vi "Create DFS Maze.vi"(10 "Height":i32, 11 "Width":i32) -> (3 "Maze":refnum<class "Maze.lvclass">)   [LabVIEW 2020, in "Maze.lvlib" / "MazeGen.lvclass"]
uses:
  MazeGen.lvclass
  Maze/Maze.lvclass
  Adjacency.ctl
  Position.ctl
  Maze.lvlib
panel:
  out "Preview":T1[][](array[typedef])
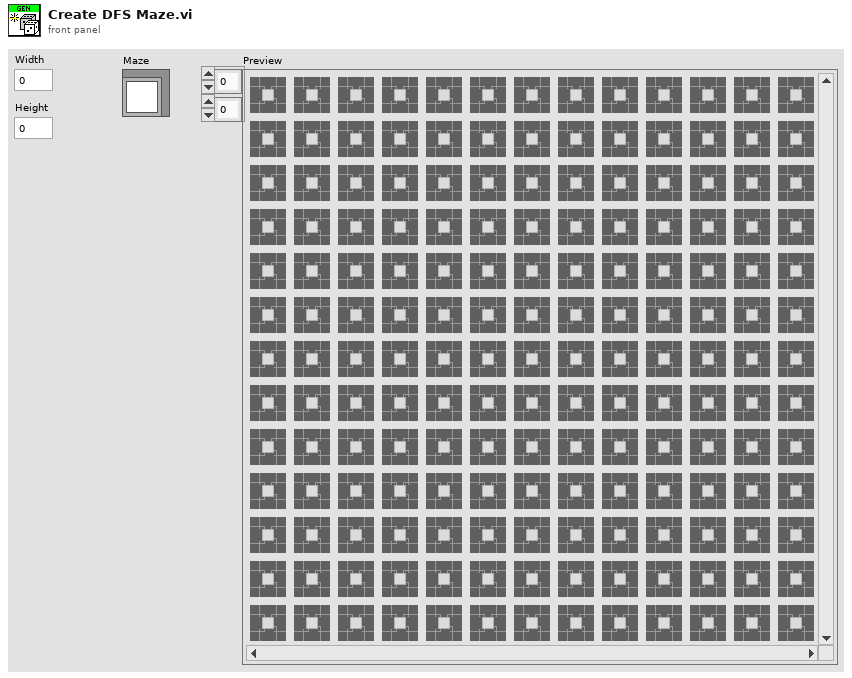
[diagram p1: front panel]
types:
  T1 = typedef "Maze.lvlib/Adjacency.ctl" = cluster{"E":bool, "N":bool, "W":bool, "S":bool, "Goal":bool, "Start":bool}
  T2 = typedef "Maze.lvlib/Position.ctl" = cluster{"S":i32, "E":i32}
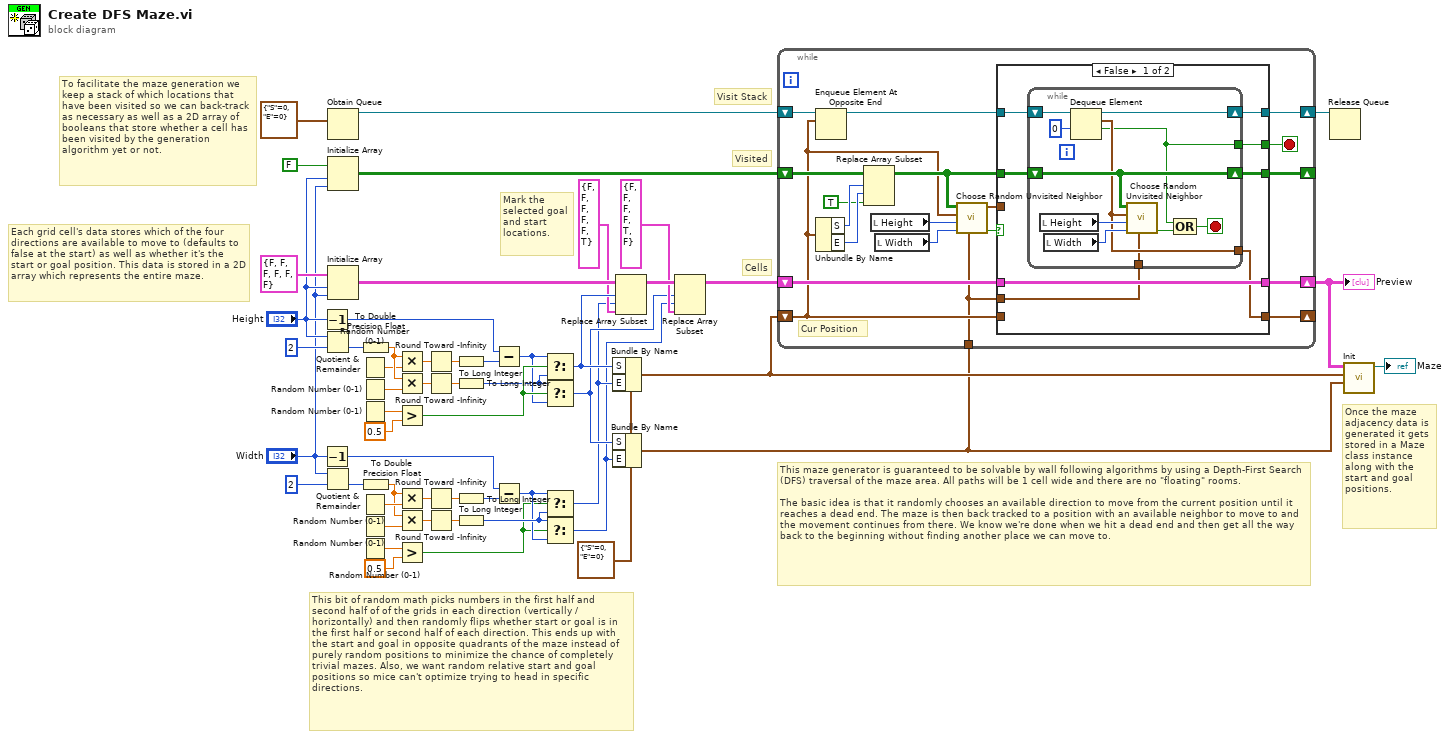
[diagram p0: block diagram]
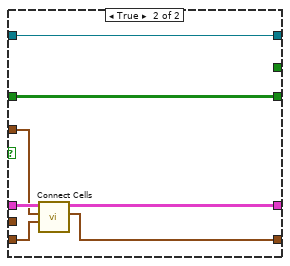
[diagram p2: hidden frame]
diagram:
  w26 = T2 {"S"=0, "E"=0} ("Position")
  # "Once the maze adjacency data is generated it gets stored in a Maze class instance along with the start and goal positions."
  # "Mark the selected goal and start locations."
  # "To facilitate the maze generation we keep a stack of which locations that have been visited so we can back-track as necessary as well as a 2D array of booleans that store whether a cell has been visited by the generation algorithm yet or not."
  # "Each grid cell's data stores which of the four directions are available to move to (defaults to false at the start) as well as whether it's the start or goal position. This data is stored in a 2D array which represents the entire maze."
  # "This maze generator is guaranteed to be solvable by wall following algorithms by using a Depth-First Search (DFS) traversal of the maze area. All paths will be 1 cell wide and there are no \"floating\" rooms.\n\nThe basic idea is that it randomly chooses an available direction to move from the current position until it reaches a dead end. The maze is then back tracked to a position with an available neighbor to move to and the movement continues from there. We know we're done when we hit a dead end and then get all the way back to the beginning without finding another place we can move to."
  # "This bit of random math picks numbers in the first half and second half of of the grids in each direction (vertically / horizontally) and then randomly flips whether start or goal is in the first half or second half of each direction. This ends up with the start and goal in opposite quadrants of the maze instead of purely random positions to minimize the chance of completely trivial mazes. Also, we want random relative start and goal positions so mice can't optimize trying to head in specific directions."
  # "Visit Stack"
  # "Visited"
  # "Cells"
  n1 = Decrement(x="Height") -> (x-1=w34:i32)
  n2 = Decrement(x="Width") -> (x-1=w44:i32)
  n3 = Quotient & Remainder(x="Height", y=2) -> (floor(x/y)=w29:i32)  [unwired: 1 out]
  n4 = Quotient & Remainder(x="Width", y=2) -> (floor(x/y)=w52:i32)  [unwired: 1 out]
  n5 = Obtain Queue(element data type=T2 {"S"=0, "E"=0} ("Position")) -> (queue out=w16:refnum<queue>)  [unwired: 4 in, 2 out]
  n6 = Initialize Array(FALSE, "Height", "Width") -> (w15:bool[][])
  n7 = Initialize Array(T1 {"E"=FALSE, "N"=FALSE, "W"=FALSE, "S"=FALSE, "Goal"=FALSE, "Start"=FALSE} ("Adjacency"), "Height", "Width") -> (w10:T1[][])
  n8 = Random Number (0-1)() -> (number: 0 to 1=w30:dbl)
  n9 = Random Number (0-1)() -> (number: 0 to 1=w31:dbl)
  n10 = Random Number (0-1)() -> (number: 0 to 1=w35:dbl)
  n11 = Random Number (0-1)() -> (number: 0 to 1=w51:dbl)
  n12 = Random Number (0-1)() -> (number: 0 to 1=w50:dbl)
  n13 = Random Number (0-1)() -> (number: 0 to 1=w43:dbl)
  n14 = To Double Precision Float(number=w29) -> (double precision float=w32:dbl)
  n15 = To Double Precision Float(number=w52) -> (double precision float=w49:dbl)
  n16 = Multiply(x=w32, y=w30) -> (x*y=w22:dbl)
  n17 = Multiply(x=w32, y=w31) -> (x*y=w21:dbl)
  n18 = Greater?(x=w35, y=0.5) -> (0:w38:bool)
  n19 = Multiply(x=w49, y=w51) -> (x*y=w24:dbl)
  n20 = Multiply(x=w49, y=w50) -> (x*y=w46:dbl)
  n21 = Greater?(x=w43, y=0.5) -> (0:w39:bool)
  n22 = Round Toward -Infinity(1:w22) -> (0:w19:dbl)
  n23 = Round Toward -Infinity(1:w21) -> (0:w20:dbl)
  n24 = Round Toward -Infinity(1:w24) -> (0:w23:dbl)
  n25 = Round Toward -Infinity(1:w46) -> (0:w25:dbl)
  n26 = To Long Integer(number=w19) -> (32bit integer=w33:i32)
  n27 = To Long Integer(number=w20) -> (32bit integer=w36:i32)
  n28 = To Long Integer(number=w23) -> (32bit integer=w45:i32)
  n29 = To Long Integer(number=w25) -> (32bit integer=w41:i32)
  n30 = Subtract(x=w34, y=w33) -> (x-y=w37:i32)
  n31 = Subtract(x=w44, y=w45) -> (x-y=w40:i32)
  n32 = Select(t=w37, s=w38, f=w36) -> (s? t:f=w9:i32)
  n33 = Select(t=w36, s=w38, f=w37) -> (s? t:f=w5:i32)
  n34 = Select(t=w40, s=w39, f=w41) -> (s? t:f=w4:i32)
  n35 = Select(t=w41, s=w39, f=w40) -> (s? t:f=w2:i32)
  n36 = Bundle By Name(cluster=w26, "S"=w9, "E"=w4) -> (w12:T2)
  n37 = Bundle By Name(cluster=w26, "S"=w5, "E"=w2) -> (w1:T2)
  n38 = Replace Array Subset(array=w10, new element=T1 {"E"=FALSE, "N"=FALSE, "W"=FALSE, "S"=FALSE, "Goal"=FALSE, "Start"=TRUE} ("new element/subarray"), index (row)=w9, index (col)=w4) -> (w7:T1[][])
  n39 = Replace Array Subset(array=w7, new element=T1 {"E"=FALSE, "N"=FALSE, "W"=FALSE, "S"=FALSE, "Goal"=TRUE, "Start"=FALSE} ("new element/subarray"), index (row)=w5, index (col)=w2) -> (w3:T1[][])
  n40 = while {
    shift-right: [w61] -> _
    shift-left: w12 -> [w57]
    shift-right: [w58] -> w14
    shift-left: w16 -> [w69]
    shift-right: [w59] -> _
    shift-left: w15 -> [w73]
    shift-right: [w60] -> w13
    shift-left: w3 -> [w62]
    tunnel: w1 -> [w55]
    stop <- w56 stop-if-true
    # "Cur Position"
    n41 = Enqueue Element At Opposite End(queue=w69, element=w57) -> (queue out=w64:refnum<queue>)  [unwired: 2 in, 2 out]
    n42 = Unbundle By Name(w57) -> ("S"=w72:i32, "E"=w71:i32)
    n43 = Replace Array Subset(array=w73, new element=TRUE ("new element/subarray"), index (row)=w72, index (col)=w71) -> (w63:bool[][])
    n44 = local read "Height"() -> (w68:i32)
    n45 = local read "Width"() -> (w67:i32)
    n46 = call "Choose Random Unvisited Neighbor.vi"("Goal"=w55, "Width"=w67, "Height"=w68, "Position"=w57, "Visited"=w63) -> ("Valid?"=w66:bool, "Random Unvisited Neighbor"=w65:T2)  [unwired: 5 in]
    n47 = case shown="False" w66 {
      tunnel: w65 -> [_ w96]
      tunnel: w64 -> [w81 w93]
      tunnel: w63 -> [w80 w94]
      tunnel: w62 -> [w76 w98]
      tunnel: w57 -> [_ w97]
      tunnel: [w75 w96] -> w61
      tunnel: [w76 w95] -> w60
      tunnel: [w77 w94] -> w59
      tunnel: [w78 w93] -> w58
      tunnel: [w79 _] -> w56
      tunnel: w55 -> [w74 _]
      frame False {
        n48 = while {
          shift-right: [w90] -> w78
          shift-left: w81 -> [w92]
          shift-right: [w89] -> w77
          shift-left: w80 -> [w89]
          tunnel: [w85] -> w79
          tunnel: [w86] -> w75
          tunnel: w74 -> [w82]
          stop <- w83 stop-if-true
          n49 = local read "Height"() -> (w88:i32)
          n50 = local read "Width"() -> (w87:i32)
          n51 = Dequeue Element(queue=w92, timeout in ms (-1)=0) -> (queue out=w90:refnum<queue>, element=w86:T2, timed out?=w85:bool)  [unwired: 1 in, 1 out]
          n52 = call "Choose Random Unvisited Neighbor.vi"("Goal"=w82, "Width"=w87, "Height"=w88, "Position"=w86, "Visited"=w89) -> ("Valid?"=w84:bool)  [unwired: 5 in, 1 out]
          n53 = Compound Arithmetic op=OR(w85, w84) -> (w83:bool)
        }
      }
      frame True {
        n54 = call "Connect Cells.vi"("To"=w97, "From"=w96, "Adjacency In"=w98) -> ("Adjacency"=w95:T1[][])  [unwired: 8 in]
      }
    }
  }
  "Preview" <- w13
  n55 = Release Queue(queue=w14) -> ()  [unwired: 2 in, 3 out]
  n56 = call "Init.vi"("Goal"=w1, "Start"=w12, "Adjacency"=w13) -> ("Maze out"=→"Maze":refnum<class "Maze.lvclass">)  [unwired: 7 in, 1 out]
